vi "GetEnumReference.vi"(8 "error in":errorcluster, 11 "Enum in":refnum<class "Enum.lvclass">) -> (0 "error out":errorcluster, 1 "Enum reference":refnum<vi>, 3 "Enum out":refnum<class "Enum.lvclass">)   [LabVIEW 2014, in "Enum.lvclass"]
uses:
  Enum.lvclass
  Generic/Generic.lvclass
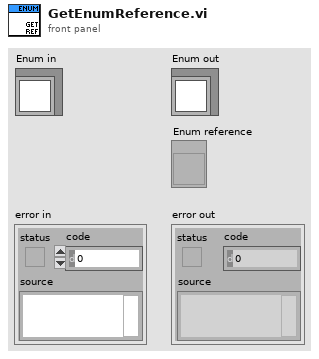
[diagram p1: front panel]
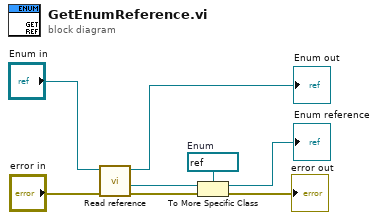
[diagram p0: block diagram]
diagram:
  w6 = refnum<vi> refnum  # Enum
  n1 = call "Read reference.vi"("error in"="error in", "GObject in"="Enum in") -> ("error out"=w7:errorcluster, "reference"=w8:refnum<vi>, "GObject out"=→"Enum out":refnum<class "Enum.lvclass">)  [unwired: 5 in]
  n2 = To More Specific Class(target class=w6, reference=w8, error in=w7) -> (specific class reference=→"Enum reference":refnum<vi>, error out=→"error out":errorcluster)
